vi "FTW-Connector-Core-Ask.vi"(0 "Actor Connector":T1, 5 "Request":string="{\"FTW-Request-Header\":\"FTW-ActorStatus\"}", 9 "Timeout":i32=100 format="%dmsec", 11 "error in":errorcluster) -> (4 "Actor Connector out":T1, 6 "Response":string, 8 "Roundtrip Time":dbl format="%.4psec", 15 "error out":errorcluster)   [LabVIEW 2015]
doc: "Performs a \"cold call\" to connect to a running Actor Instance at the given Instance Inbox Address. Normally, this method is wrapped by a \"Construct\" method in each specific Actor Connector subclass."
uses:
  core/type/FTW-Type-Actor-Connector.ctl
  json/FTW-JSON-Type.ctl
  error/FTW-ERR-NoErrorConstant.vi
panel:
  # "Inputs"
  # "Outputs"
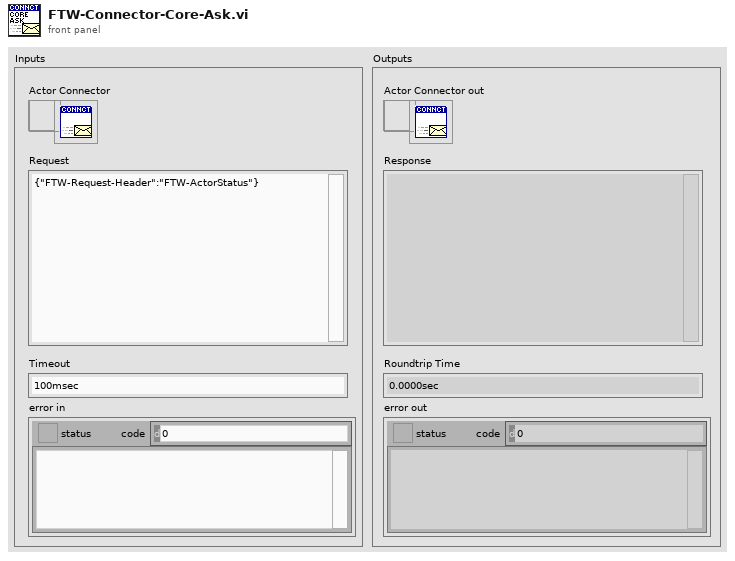
[diagram p1: front panel]
types:
  T1 = typedef "FTW-Type-Actor-Connector.ctl" = refnum<data-value>
  T2 = typedef "FTW-JSON-Type.ctl" = enum8{"Not Found", "Object", "Array", "String", "Number", "Boolean", "null"}
  T3 = typedef "FTW-Type-JSON.ctl" = refnum<data-value>
  T4 = cluster{"FTW-CodeGen-Type":enum16{"FTW-Actor-Connector"}, "Socket":i64}
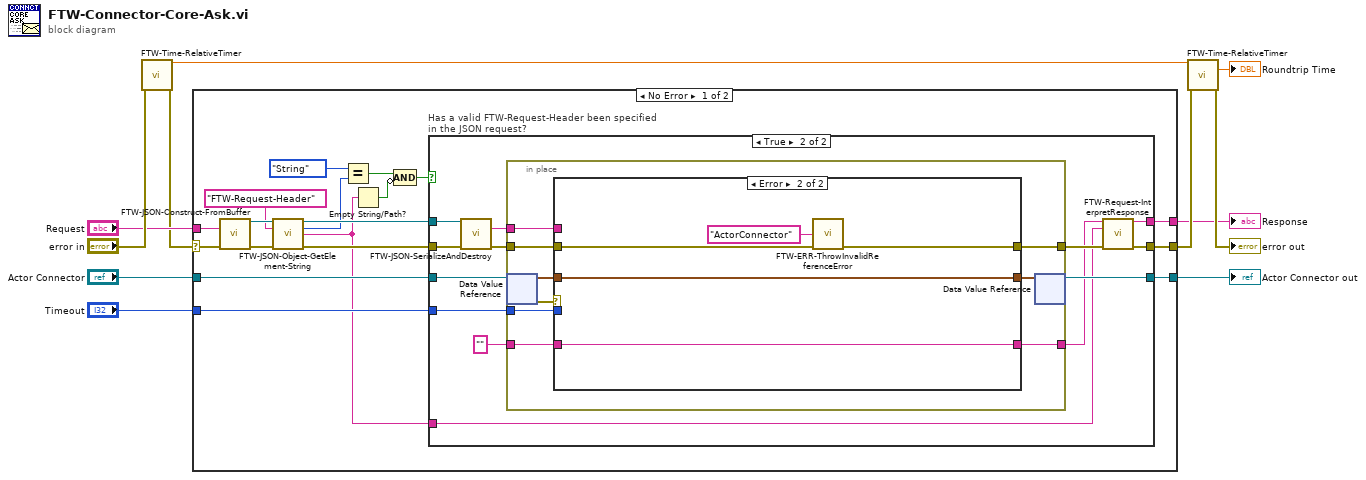
[diagram p0: block diagram]
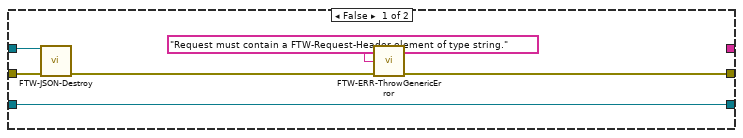
[diagram p2: hidden frame]
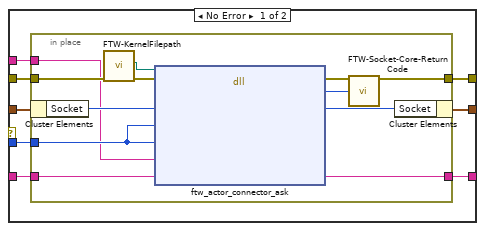
[diagram p3: hidden frame]
diagram:
  n1 = call "FTW-Time-RelativeTimer.vi"("error in"="error in") -> ("Current Timer Value"=w7:dbl, "error out"=w1:errorcluster)  [unwired: 12 in, 1 out]
  n2 = case shown="No Error" w1 {
    selector: w1 -> [w12 w83]
    tunnel: "Actor Connector" -> [w29 w84]
    tunnel: [w28 w84] -> w10
    tunnel: "Timeout" -> [w27 _]
    tunnel: [w26 w83] -> w4
    tunnel: [w16 _] -> w3
    tunnel: "Request" -> [w14 _]
    frame No Error {
      n3 = call "FTW-JSON-Construct-FromBuffer.vi"("JSON String (UTF-8)"=w14, "error in"=w12) -> ("JSON"=w25:T3, "error out"=w24:errorcluster)  [unwired: 12 in]
      n4 = call "FTW-JSON-Object-GetElement-String.vi"("JSON"=w25, "Key"="FTW-Request-Header", "error in"=w24) -> ("JSON out"=w23:T3, "JSON Element Type"=w20:T2, "Value"=w15:string, "error out"=w22:errorcluster)  [unwired: 9 in]
      n5 = Equal?(x=FTW-JSON-Type."String" ("JSON Element Type"), y=w20) -> (x = y?=w19:bool)
      n6 = Empty String/Path?(string/path=w15) -> (empty?=w18:bool)
      n7 = Compound Arithmetic op=AND(w19, invert w18) -> (w13:bool)
      n8 = case "Has a valid FTW-Request-Header been specified in the JSON request?" shown="True" w13 {
        tunnel: w29 -> [w35 w47]
        tunnel: [w35 w46] -> w28
        tunnel: w27 -> [_ w45]
        tunnel: [w30 w44] -> w26
        tunnel: w23 -> [w34 w43]
        tunnel: w22 -> [w33 w42]
        tunnel: [_ w40] -> w16
        tunnel: w15 -> [_ w39]
        frame False {
          n9 = call "FTW-JSON-Destroy.vi"("JSON"=w34, "error in"=w33) -> ("error out"=w31:errorcluster)  [unwired: 13 in]
          n10 = call "FTW-ERR-ThrowGenericError.vi"("Error Message"="Request must contain a FTW-Request-Header element of type string.", "error in"=w31) -> ("error out"=w30:errorcluster)  [unwired: 13 in]
        }
        frame True {
          n11 = call "FTW-JSON-SerializeAndDestroy.vi"("JSON"=w43, "error in"=w42) -> ("JSON String (UTF-8)"=w38:string, "error out"=w41:errorcluster)  [unwired: 12 in]
          n12 = in-place {
            in-place-border: w41 -> [w57]
            in-place-border: [w56] -> w48
            in-place-border: [w55] -> w37
            in-place-border: w45 -> [w54]
            in-place-border: w38 -> [w53]
            in-place-border: "" -> [w49]
            n13 = in-place-dvr #1(w47) -> (w52:T4, w50:errorcluster)
            n14 = case shown="Error" w50 {
              tunnel: w57 -> [w65 w79]
              tunnel: [w64 w78] -> w56
              tunnel: [w63 w81] -> w55
              tunnel: w54 -> [w62 _]
              tunnel: w53 -> [w61 _]
              tunnel: w52 -> [w60 w82]
              tunnel: [w59 w82] -> w51
              tunnel: w49 -> [w58 w81]
              frame No Error {
                n15 = in-place {
                  in-place-border: w65 -> [w72]
                  in-place-border: [w69] -> w64
                  in-place-border: [w66] -> w63
                  in-place-border: w62 -> [w71]
                  in-place-border: w61 -> [w70]
                  in-place-border: w58 -> [w68]
                  n16 = in-place-cluster #2(w60) -> ("Socket"=w76:i64)
                  n17 = call "FTW-KernelFilepath.vi"("error in"=w72) -> ("error out"=w74:errorcluster, "Library Filepath"=w73:path)  [unwired: 8 in, 1 out]
                  n18 = dll-call lib="?" fn="ftw_actor_connector_ask"(path in=w73, error in=w74, "Socket Handle"=w76, "Send Timeout"=w71, "Recv Timeout"=w71, "Request"=w70, "Response"=w68) -> (error out=w77:errorcluster, "Return Code"=w67:i64, "Socket Handle"=w75:i64, "Response"=w66:string)  [unwired: 4 in, 1 out]
                  n19 = call "FTW-Socket-Core-ReturnCode.vi"("error in"=w77, "Return Code"=w67) -> ("error out"=w69:errorcluster)  [unwired: 13 in]
                  n20 = in-place-cluster #2("Socket"=w75) -> (w59:T4)
                }
              }
              frame Error {
                n21 = call "FTW-ERR-ThrowInvalidReferenceError.vi"("Reference Type"="ActorConnector", "error in"=w79) -> ("error out"=w78:errorcluster)  [unwired: 13 in]
              }
            }
            n22 = in-place-dvr #1(w51) -> (w46:T1)  [unwired: 1 out]
          }
          n23 = call "FTW-Request-InterpretResponse.vi"("Raw Response"=w37, "Expected Request Header"=w39, "error in"=w48) -> ("JSON Response"=w40:string, "error out"=w44:errorcluster)  [unwired: 11 in]
        }
      }
    }
    frame Error {
    }
  }
  "Actor Connector out" <- w10
  "Response" <- w3
  n24 = call "FTW-Time-RelativeTimer.vi"("Previous Timer Value"=w7, "error in"=w4) -> ("Elapsed Time"=→"Roundtrip Time":dbl, "error out"=→"error out":errorcluster)  [unwired: 11 in, 1 out]
